vi "Execution_StartExternalProcess.vi"(8 "error in (no error)":errorcluster, 9 "ProcessConfig":T1={"Path"=path "", "Timeout"=0.0, "viInitString"="", "State"=enum."Closed"}, 10 "Process in":refnum<class "Process.lvclass">, 11 "EVE reference in":refnum<data-value>) -> (0 "error out":errorcluster, 3 "EVE reference out":refnum<data-value>)   [LabVIEW 2013, in "Process.lvclass"]
uses:
  Process.lvclass
  050 - CONFIG/20 - ExternalProcesses/paramsExternalProcesses.ctl
  001 - MAIN/Class/EVE/EVE.lvclass
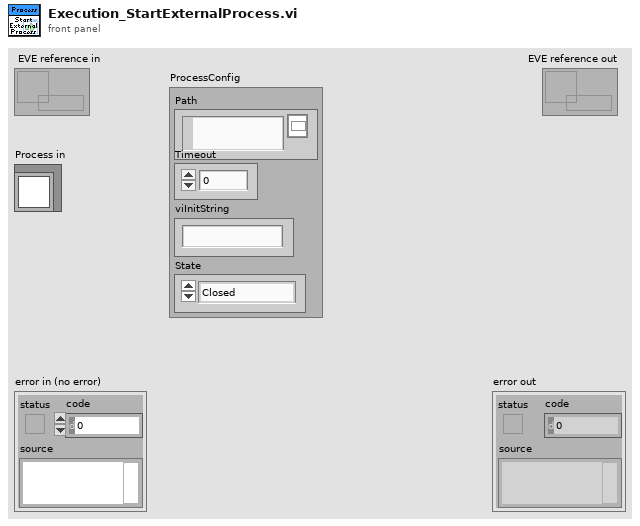
[diagram p1: front panel]
types:
  T1 = typedef "paramsExternalProcesses.ctl" = cluster{"Path":path, "Timeout":dbl, "viInitString":string, "State":enum32{"Invalid", "Standard", "Closed", "Hidden", "Minimized", "Maximized"}}
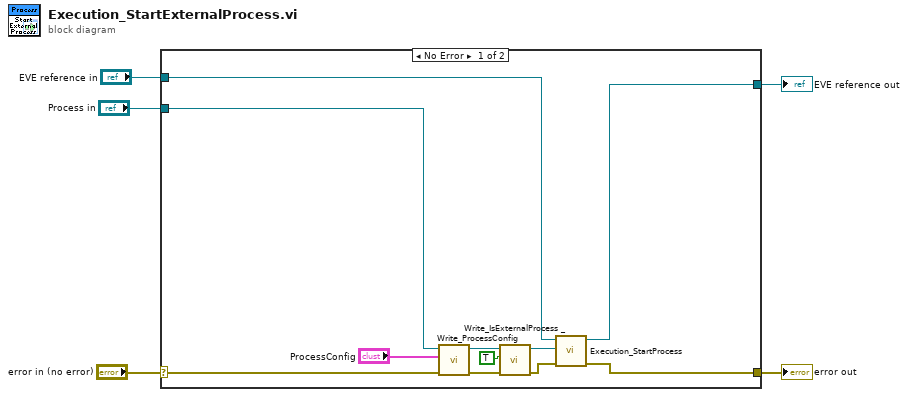
[diagram p0: block diagram]
diagram:
  n1 = case shown="No Error" "error in (no error)" {
    selector: "error in (no error)" -> [w11 w18]
    tunnel: [w10 w18] -> w4
    tunnel: "Process in" -> [w9 _]
    tunnel: "EVE reference in" -> [w8 w17]
    tunnel: [w7 w17] -> w1
    frame No Error {
      n2 = call-dynamic "Write_ProcessConfig.vi"("error in (no error)"=w11, "ProcessConfig"="ProcessConfig", "Process in"=w9) -> ("error out"=w12:errorcluster, "Process out"=w13:refnum<class "Process.lvclass">)  [unwired: 7 in]
      n3 = call-dynamic "Write_IsExternalProcess _.vi"("error in (no error)"=w12, "ExternalProcess ?"=TRUE, "Process in"=w13) -> ("error out"=w15:errorcluster, "Process out"=w16:refnum<class "Process.lvclass">)  [unwired: 7 in]
      n4 = call "Execution_StartProcess.vi"("error in (no error)"=w15, "Process in"=w16, "EVE reference in"=w8) -> ("error out"=w10:errorcluster, "EVE reference out"=w7:refnum<data-value>)  [unwired: 7 in]
    }
    frame Error {
    }
  }
  "error out" <- w4
  "EVE reference out" <- w1
